vi "test1.vi"() -> ()   [LabVIEW 2020]
panel:
  in  "stop":bool
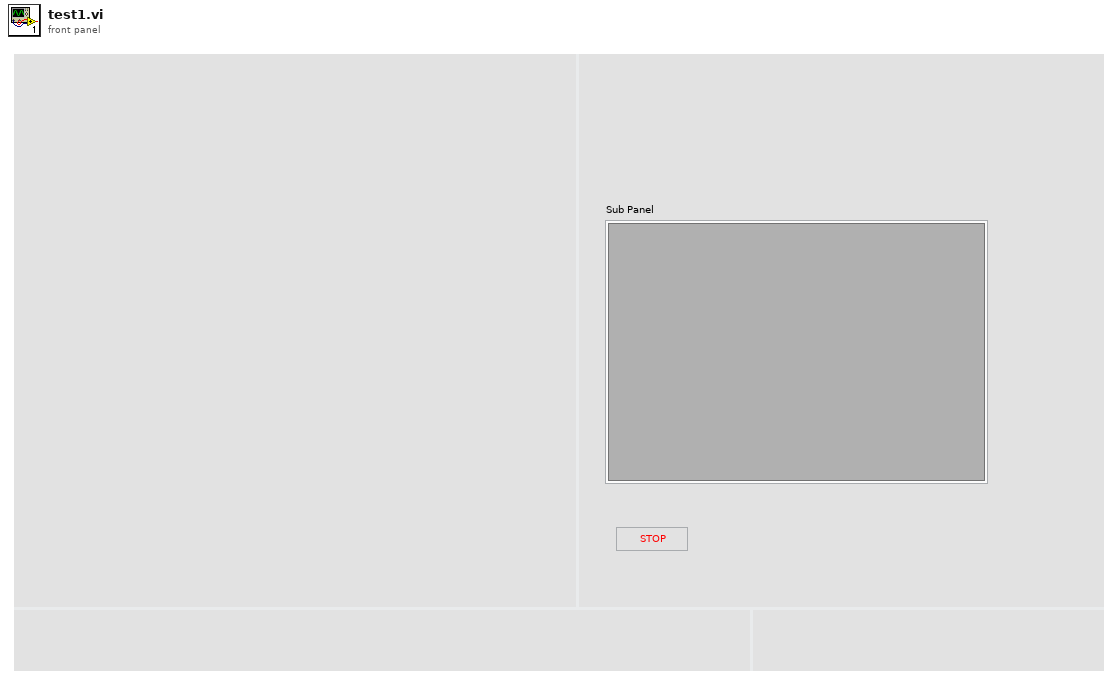
[diagram p1: front panel]
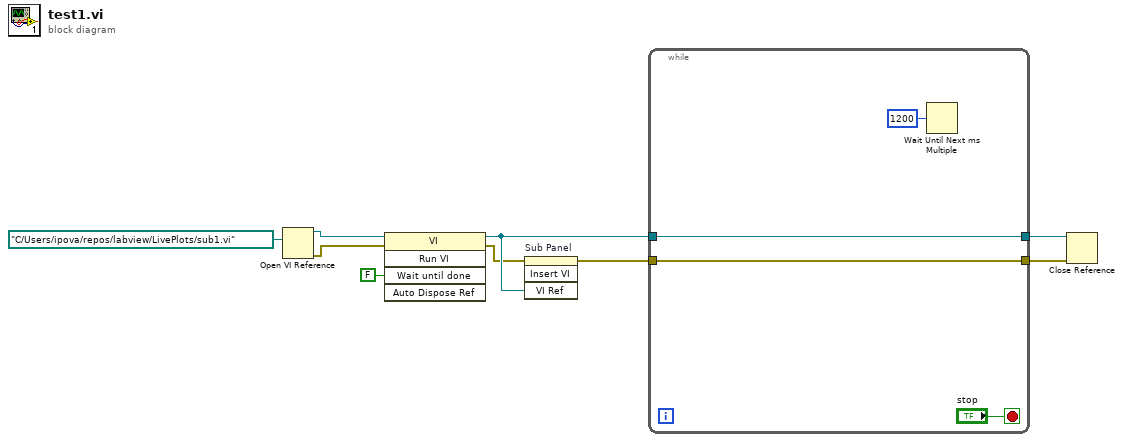
[diagram p0: block diagram]
diagram:
  n1 = Open VI Reference(vi path=path "C:/Users/ipova/repos/labview/LivePlots/sub1.vi") -> (vi reference=w8:refnum<vi>, error out=w4:errorcluster)  [unwired: 5 in]
  n2 = invoke class="VI" method="Run VI"(reference=w8, error in=w4, "Wait until done"=FALSE ("Wait Until Done")) -> (reference out=w6:refnum<vi>, error out=w3:errorcluster)  [unwired: 2 in, 3 out]
  n3 = invoke on="Sub Panel" class="SubPnl" method="Insert VI"(error in=w3, "VI Ref"=w6) -> (error out=w2:errorcluster)  [unwired: 2 in, 3 out]
  n4 = while {
    tunnel: w6 -> [w11]
    tunnel: [w11] -> w5
    tunnel: w2 -> [w10]
    tunnel: [w10] -> w1
    stop <- "stop" stop-if-true
    n5 = Wait Until Next ms Multiple(millisecond multiple=u32 1200) -> ()  [unwired: 1 out]
  }
  n6 = Close Reference(reference=w5, error in (no error)=w1) -> ()  [unwired: 1 out]
